vi "Read Page General Properties.vi"(8 "Error In":errorcluster, 11 "Custom Device Page .NET Ref In":refnum<k24>) -> (0 "Error Out":errorcluster, 2 "General Page Properties":T3, 3 "Custom Device Page .NET Ref Out":refnum<k24>)   [LabVIEW 2015, in "VeriStand Custom Device XML Parser.lvlib"]
doc: "Reads and returns the general properties of the page"
uses:
  VeriStand Custom Device XML Parser.lvlib
  NationalInstruments.VeriStand.XMLReader
  XML Controls/Path Cluster.ctl
  XML Controls/Help File Properties.ctl
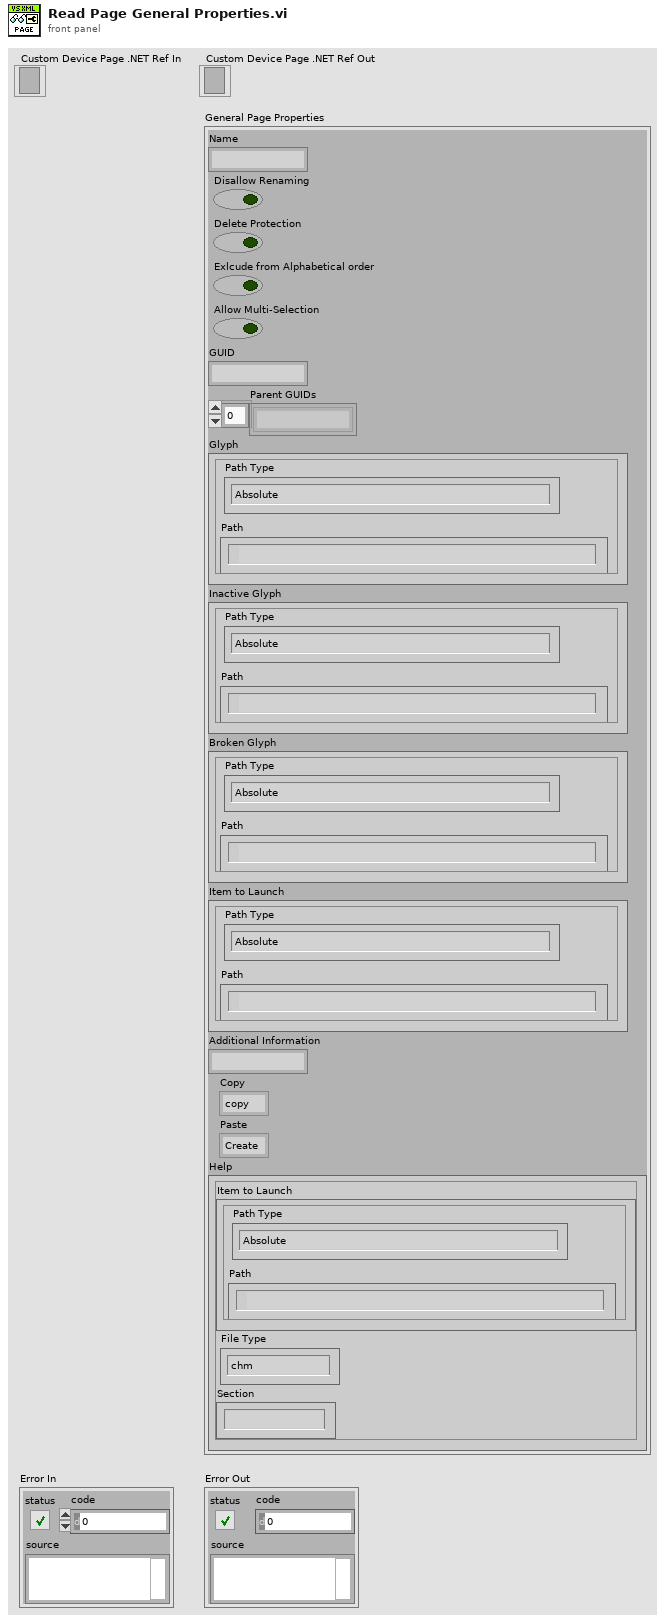
[diagram p1: front panel]
types:
  T1 = typedef "VeriStand Custom Device XML Parser.lvlib/Path Cluster.ctl" = cluster{"Path":path, "Path Type":enum16{"Absolute", "To Base", "To Common Doc Dir", "To Application Data Dir"}}
  T2 = typedef "VeriStand Custom Device XML Parser.lvlib/Help File Properties.ctl" = cluster{"Item to Launch":T1, "Section":string, "File Type":enum16{"chm", "other"}}
  T3 = cluster{"Name":string, "Disallow Renaming":bool, "Delete Protection":bool, "Exlcude from Alphabetical order":bool, "Allow Multi-Selection":bool, "GUID":string, "Parent GUIDs":string[], "Glyph":T1, "Inactive Glyph":T1, "Broken Glyph":T1, "Item to Launch":T1, "Additional Information":string, "Copy":enum16{"copy", "disabled"}, "Paste":enum16{"Create", "CreatIfNotExists_GUID", "CreatIfNotExists_Name", "Replace", "Dialog"}, "Help":T2}
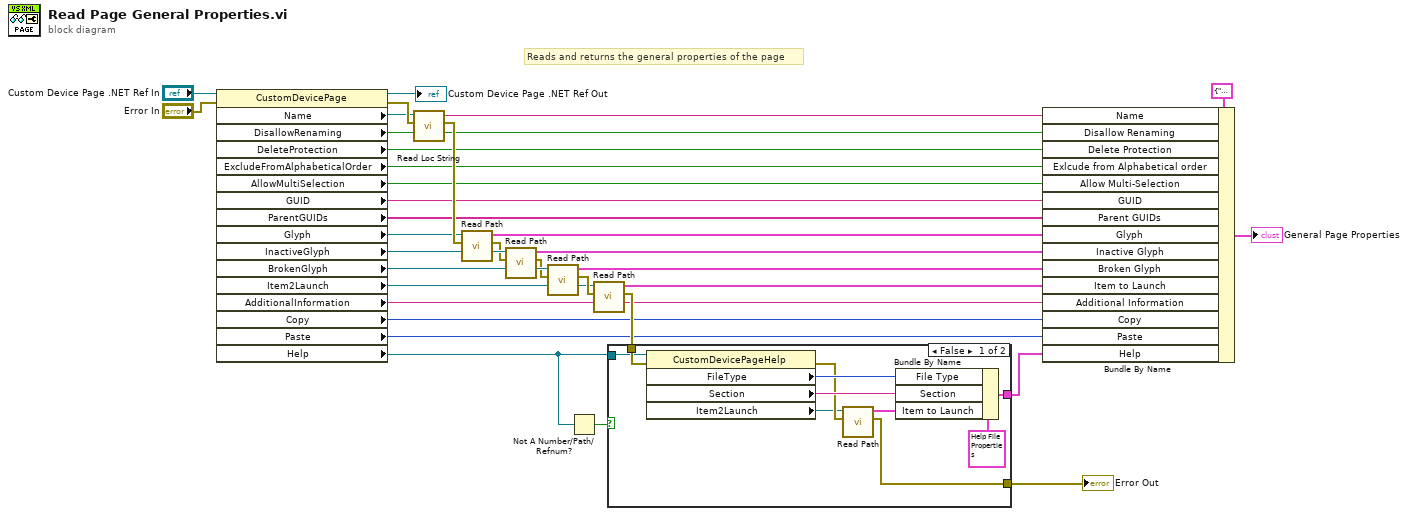
[diagram p0: block diagram]
diagram:
  # "Reads and returns the general properties of the page"
  n1 = property class="CustomDevicePage"(reference="Custom Device Page .NET Ref In", error in="Error In") -> (reference out=→"Custom Device Page .NET Ref Out":refnum<k24>, error out=w7:errorcluster, "Name"=w6:refnum<k24>, "DisallowRenaming"=w9:bool, "DeleteProtection"=w10:bool, "ExcludeFromAlphabeticalOrder"=w11:bool, "AllowMultiSelection"=w12:bool, "GUID"=w13:string, "ParentGUIDs"=w14:string[], "Glyph"=w15:refnum<k24>, "InactiveGlyph"=w19:refnum<k24>, "BrokenGlyph"=w20:refnum<k24>, "Item2Launch"=w21:refnum<k24>, "AdditionalInformation"=w23:string, "Copy"=w28:i32, "Paste"=w29:i32, "Help"=w1:refnum<k24>)
  n2 = call "Read Loc String.vi"("Error In"=w7, "Loc String .NET Ref"=w6) -> ("Error Out"=w16:errorcluster, "English"=w8:string)  [unwired: 7 in, 1 out]
  n3 = call "Read Path.vi"("Error In"=w16, "Path .NET Ref"=w15) -> ("Error Out"=w17:errorcluster, "Path Properties"=w24:T1)  [unwired: 8 in]
  n4 = call "Read Path.vi"("Error In"=w17, "Path .NET Ref"=w19) -> ("Error Out"=w18:errorcluster, "Path Properties"=w25:T1)  [unwired: 8 in]
  n5 = call "Read Path.vi"("Error In"=w18, "Path .NET Ref"=w20) -> ("Error Out"=w22:errorcluster, "Path Properties"=w26:T1)  [unwired: 8 in]
  n6 = Not A Number/Path/Refnum?(number/path/refnum=w1) -> (NaN/Path/Refnum?=w2:bool)
  n7 = call "Read Path.vi"("Error In"=w22, "Path .NET Ref"=w21) -> ("Error Out"=w30:errorcluster, "Path Properties"=w27:T1)  [unwired: 8 in]
  n8 = case shown="False" w2 {
    tunnel: [w44 w45] -> w32
    tunnel: [w43 _] -> w31
    tunnel: w30 -> [w37 w45]
    tunnel: w1 -> [w36 _]
    frame False {
      n9 = property class="CustomDevicePageHelp"(reference=w36, error in=w37) -> (error out=w39:errorcluster, "FileType"=w40:i32, "Section"=w41:string, "Item2Launch"=w38:refnum<k24>)  [unwired: 1 out]
      n10 = call "Read Path.vi"("Error In"=w39, "Path .NET Ref"=w38) -> ("Error Out"=w44:errorcluster, "Path Properties"=w42:T1)  [unwired: 8 in]
      n11 = Bundle By Name(cluster=T2 {"Item to Launch"={"Path"=path "", "Path Type"=enum."Absolute"}, "Section"="", "File Type"=enum."chm"} ("Help"), "File Type"=w40, "Section"=w41, "Item to Launch"=w42) -> (w43:T2)
    }
    frame True {
    }
  }
  "Error Out" <- w32
  n12 = Bundle By Name(cluster=T3 {"Name"="", "Disallow Renaming"=FALSE, "Delete Protection"=FALSE, "Exlcude from Alphabetical order"=FALSE, "Allow Multi-Selection"=FALSE, "GUID"="", "Parent GUIDs"=[], "Glyph"={"Path"=path "", "Path Type"=enum."Absolute"}, "Inactive Glyph"={"Path"=path "", "Path Type"=enum."Absolute"}, "Broken Glyph"={"Path"=path "", "Path Type"=enum."Absolute"}, "Item to Launch"={"Path"=path "", "Path Type"=enum."Absolute"}, "Additional Information"="", "Copy"=enum."copy", "Paste"=enum."Create", "Help"={"Item to Launch"={"Path"=path "", "Path Type"=enum."Absolute"}, "Section"="", "File Type"=enum."chm"}}, "Name"=w8, "Disallow Renaming"=w9, "Delete Protection"=w10, "Exlcude from Alphabetical order"=w11, "Allow Multi-Selection"=w12, "GUID"=w13, "Parent GUIDs"=w14, "Glyph"=w24, "Inactive Glyph"=w25, "Broken Glyph"=w26, "Item to Launch"=w27, "Additional Information"=w23, "Copy"=w28, "Paste"=w29, "Help"=w31) -> (→"General Page Properties":T3)
